vi "Merge Image.vi"(8 "error in (no error)":errorcluster, 10 "Camera Control Cluster":T1={"Core"={"Current VI Reference"=refnum, "Close Panel on Exit?"=FALSE}, "CC ID"=0, "Part name"="", "Number of active cameras"=[], "IA Camera names"=[], "Image count array"=[], "Diagnostics Child ID"=-1, "Number of cameras"=0, "Image array"=[], "LiveMode"=TRUE, "RecieversID"=[], "Active Camera ID"=[], "Enqueuer"={"Caller Enqueuer"=refnum, "Nested Actor's Enqueuer"=[], "Reciever Enqueuer "=[]}, "Image Array Counter"=0, "Images Recieved count"=[], "All Camera Diagnostics"=FALSE, "Output Data"={"Launch Handshake"={"Actor Enqueuer Refnum"=refnum, "Actor core Refnum"=refnum, "Actor Name"=""}, "Launch Clear"=TRUE, "Part Name"="", "Image Trigger Count"=0, "Image Array"=[], "CamOpticsDiagnosticsResult"={"Light Camera  Name"="", "Diagnosed Image"=refnum, "Dust Percentage"=0.0, "Result"=FALSE}, "State Ack"={"State Message"="", "Status"=""}, "Error Handler"="", "Camera Information"=[], "Number of Active Camera"=0}, "Camera Setup"=[], "Setup Response Received Count"=0, "Send Error to Caller"=FALSE, "Camera Info Recieved"=0, "CameraControllerParameters"={"CameraControllerParameters"={"ID"=0, "FrontPanelOpen"=FALSE, "NoOfCameras"=0, "CameraID"=[], "NoOfReceivers"=0, "Diagnostics"={"Path"="", "LightCameraSequence"=[], "Delaytime"=0.0, "DecisitionParameters"={"Range"=[], "AcceptancePercentage"=[], "Comparison"=[], "AcceptableBlackBinValue"=0}, "DiagnosticReceiverSequence"={"ReceiverName"="", "ReceiverID"=0}}, "PartsList"=[]}, "PartName"=[]}, "CurrentPartDetails"={"PartName"="", "CameraIDs"=[], "ReceiverSequence"=[]}, "Run Info"={"State"="", "Image File path"=[]}, "Active Light Camera Name"="", "Captured Image Info"={"Image out"=refnum, "Camera Location"="", "Count"=0, "RecieverSequence"=[{"RecieverID"=0.0, "Index"=1.0}, {"RecieverID"=1.0, "Index"=2.0}]}, "Current Steps"="", "CurrentReceiverSequence"=[], "Status Ack"=[]}, 11 "Camera Controller in":refnum<class "Camera Controller.lvclass">) -> (0 "error out":errorcluster, 2 "Camera Control Cluster Out":T1={"Core"={"Current VI Reference"=refnum, "Close Panel on Exit?"=FALSE}, "CC ID"=0, "Part name"="", "Number of active cameras"=[], "IA Camera names"=[], "Image count array"=[], "Diagnostics Child ID"=-1, "Number of cameras"=0, "Image array"=[], "LiveMode"=TRUE, "RecieversID"=[], "Active Camera ID"=[], "Enqueuer"={"Caller Enqueuer"=refnum, "Nested Actor's Enqueuer"=[], "Reciever Enqueuer "=[]}, "Image Array Counter"=0, "Images Recieved count"=[], "All Camera Diagnostics"=FALSE, "Output Data"={"Launch Handshake"={"Actor Enqueuer Refnum"=refnum, "Actor core Refnum"=refnum, "Actor Name"=""}, "Launch Clear"=TRUE, "Part Name"="", "Image Trigger Count"=0, "Image Array"=[], "CamOpticsDiagnosticsResult"={"Light Camera  Name"="", "Diagnosed Image"=refnum, "Dust Percentage"=0.0, "Result"=FALSE}, "State Ack"={"State Message"="", "Status"=""}, "Error Handler"="", "Camera Information"=[], "Number of Active Camera"=0}, "Camera Setup"=[], "Setup Response Received Count"=0, "Send Error to Caller"=FALSE, "Camera Info Recieved"=0, "CameraControllerParameters"={"CameraControllerParameters"={"ID"=0, "FrontPanelOpen"=FALSE, "NoOfCameras"=0, "CameraID"=[], "NoOfReceivers"=0, "Diagnostics"={"Path"="", "LightCameraSequence"=[], "Delaytime"=0.0, "DecisitionParameters"={"Range"=[], "AcceptancePercentage"=[], "Comparison"=[], "AcceptableBlackBinValue"=0}, "DiagnosticReceiverSequence"={"ReceiverName"="", "ReceiverID"=0}}, "PartsList"=[]}, "PartName"=[]}, "CurrentPartDetails"={"PartName"="", "CameraIDs"=[], "ReceiverSequence"=[]}, "Run Info"={"State"="", "Image File path"=[]}, "Active Light Camera Name"="", "Captured Image Info"={"Image out"=refnum, "Camera Location"="", "Count"=0, "RecieverSequence"=[{"RecieverID"=0.0, "Index"=1.0}, {"RecieverID"=1.0, "Index"=2.0}]}, "Current Steps"="", "CurrentReceiverSequence"=[], "Status Ack"=[]}, 3 "Camera Controller out":refnum<class "Camera Controller.lvclass">)   [LabVIEW 2019, in "Camera Controller.lvlib" / "Camera Controller.lvclass"]
uses:
  Camera Controller.lvclass
  <vilib>/vision/Image Controls.llb/IMAQ Image.ctl
  <vilib>/ActorFramework/Actor/Actor.lvclass
  Image Trigger Global Count.vi
  C:/Program Files/National Instruments/LabVIEW 2019/vi.lib/ActorFramework/Actor/Actor.lvclass
  <vilib>/ActorFramework/Message Enqueuer/Message Enqueuer.lvclass
  TypeDef/Output Data.ctl
  TypeDef/CameraControllerParameters.ctl
  TypeDef/Initialize Data CC.ctl
panel:
  out "min value":i32
  out "output array":T2[][](array[typedef])
  in  "appended array in":T2[][](array[typedef])
  out "appended array out":T2[][](array[typedef])
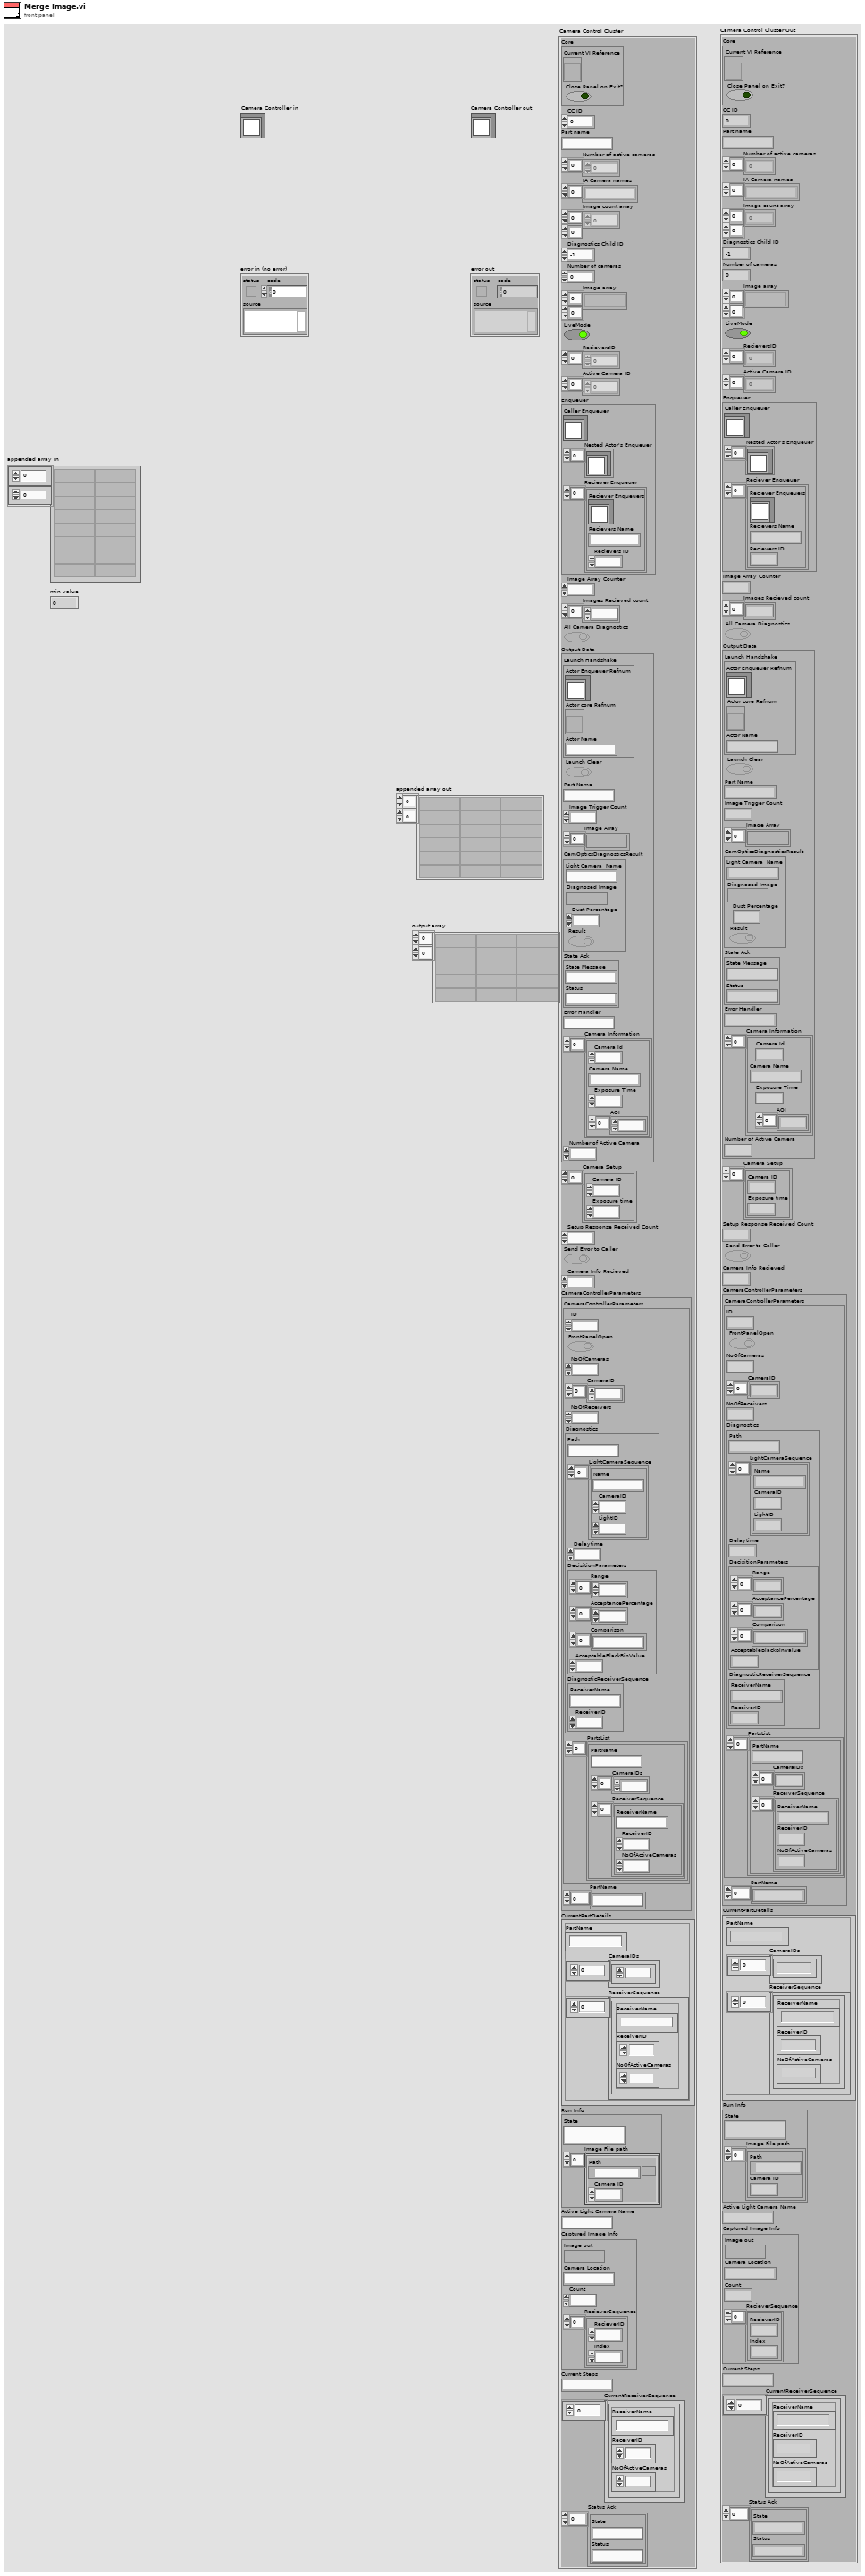
[diagram p1: front panel]
types:
  T1 = typedef "Camera Controller.lvlib/Camera Controller.lvclass/Initialize Data CC.ctl" = cluster{"Core":cluster{"Current VI Reference":refnum<vi>, "Close Panel on Exit?":bool}, "CC ID":i32, "Part name":string, "Number of active cameras":i32[], "IA Camera names":string[], "Image count array":i32[][], "Diagnostics Child ID":i32, "Number of cameras":i32, "Image array":T2[][], "LiveMode":bool, "RecieversID":i32[], "Active Camera ID":i32[], "Enqueuer":cluster{"Caller Enqueuer":refnum<class "Message Enqueuer.lvclass">, "Nested Actor's Enqueuer":refnum<class "Message Enqueuer.lvclass">[], "Reciever Enqueuer ":cluster{"Reciever Enqueuers":refnum<class "Message Enqueuer.lvclass">, "Recievers Name":string, "Recievers ID":i32}[]}, "Image Array Counter":u64, "Images Recieved count":u64[], "All Camera Diagnostics":bool, "Output Data":T3, "Camera Setup":cluster{"Camera ID":i32, "Exposure time":i32}[], "Setup Response Received Count":u64, "Send Error to Caller":bool, "Camera Info Recieved":i32, "CameraControllerParameters":T4, "CurrentPartDetails":cluster{"PartName":string, "CameraIDs":i32[], "ReceiverSequence":cluster{"ReceiverName":string, "ReceiverID":i32, "NoOfActiveCameras":i32}[]}, "Run Info":cluster{"State":string, "Image File path":cluster{"Path":path, "Camera ID":i32}[]}, "Active Light Camera Name":string, "Captured Image Info":cluster{"Image out":T2, "Camera Location":string, "Count":u64, "RecieverSequence":cluster{"RecieverID":dbl, "Index":dbl}[]}, "Current Steps":string, "CurrentReceiverSequence":cluster{"ReceiverName":string, "ReceiverID":i32, "NoOfActiveCameras":i32}[], "Status Ack":cluster{"State":string, "Status":string}[]}
  T2 = typedef "IMAQ Image.ctl" = refnum<image>
  T3 = typedef "Camera Controller.lvlib/Camera Controller.lvclass/Output Data.ctl" = cluster{"Launch Handshake":cluster{"Actor Enqueuer Refnum":refnum<class "Message Enqueuer.lvclass">, "Actor core Refnum":refnum<vi>, "Actor Name":string}, "Launch Clear":bool, "Part Name":string, "Image Trigger Count":u64, "Image Array":T2[], "CamOpticsDiagnosticsResult":cluster{"Light Camera  Name":string, "Diagnosed Image":T2, "Dust Percentage":dbl, "Result":bool}, "State Ack":cluster{"State Message":string, "Status":string}, "Error Handler":string, "Camera Information":cluster{"Camera Id":i32, "Camera Name":string, "Exposure Time":i32, "AOI":i32[]}[], "Number of Active Camera":i32}
  T4 = typedef "Camera Controller.lvlib/Camera Controller.lvclass/CameraControllerParameters.ctl" = cluster{"CameraControllerParameters":cluster{"ID":i32, "FrontPanelOpen":bool, "NoOfCameras":i32, "CameraID":i32[], "NoOfReceivers":i32, "Diagnostics":cluster{"Path":string, "LightCameraSequence":cluster{"Name":string, "CameraID":i32, "LightID":i32}[], "Delaytime":dbl, "DecisitionParameters":cluster{"Range":i32[], "AcceptancePercentage":i32[], "Comparison":string[], "AcceptableBlackBinValue":i32}, "DiagnosticReceiverSequence":cluster{"ReceiverName":string, "ReceiverID":i32}}, "PartsList":cluster{"PartName":string, "CameraIDs":i32[], "ReceiverSequence":cluster{"ReceiverName":string, "ReceiverID":i32, "NoOfActiveCameras":i32}[]}[]}, "PartName":string[]}
  T5 = cluster{"ReceiverName":string, "ReceiverID":i32, "NoOfActiveCameras":i32}[]
  T6 = cluster{"ReceiverName":string, "ReceiverID":i32, "NoOfActiveCameras":i32}
  T7 = cluster{"Reciever Enqueuers":refnum<class "Message Enqueuer.lvclass">, "Recievers Name":string, "Recievers ID":i32}[]
  T8 = cluster{"Reciever Enqueuers":refnum<class "Message Enqueuer.lvclass">, "Recievers Name":string, "Recievers ID":i32}
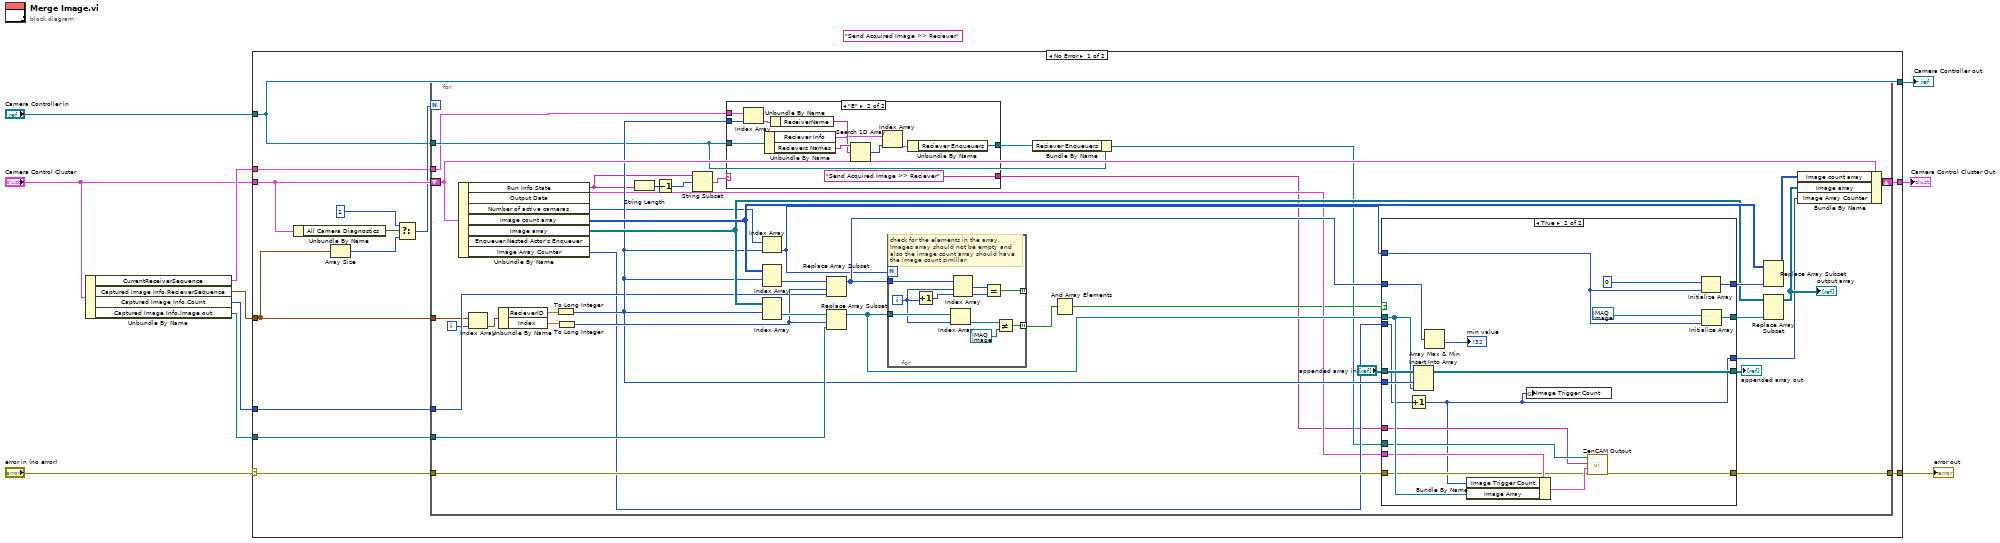
[diagram p0: block diagram]
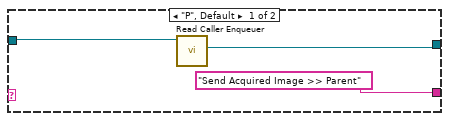
[diagram p2: hidden frame]
diagram:
  (unwired) "Send Acquired Image >> Reciever" ("State")
  n1 = Unbundle By Name("Camera Control Cluster") -> ("CurrentReceiverSequence"=w8:T5, "Captured Image Info.RecieverSequence"=w7:cluster{"RecieverID":dbl, "Index":dbl}[], "Captured Image Info.Count"=w6:u64, "Captured Image Info.Image out"=w5:T2)
  n2 = case shown="No Error" "error in (no error)" {
    selector: "error in (no error)" -> [w21 w114]
    tunnel: w7 -> [w17 _]
    tunnel: w6 -> [w23 _]
    tunnel: w5 -> [w15 _]
    tunnel: "Camera Control Cluster" -> [w19 w115]
    tunnel: [w22 w115] -> w2
    tunnel: [w20 w114] -> w3
    tunnel: w8 -> [w12 _]
    tunnel: "Camera Controller in" -> [w11 w113]
    tunnel: [w11 w113] -> w1
    frame No Error {
      n3 = Unbundle By Name(w19) -> ("All Camera Diagnostics"=w16:bool)
      n4 = Array Size(array=w17) -> (size(s)=w13:i32)
      n5 = Select(t=1 ("f"), s=w16, f=w13) -> (s? t:f=w18:i32)
      n6 = for {
        N: w18 -> [_]
        tunnel: w23 -> [w44]
        tunnel: w15 -> [w59]
        shift-right: [w50] -> w22
        shift-left: w19 -> [w57]
        tunnel: w21 -> [w45]
        tunnel: [w46] -> w20
        tunnel: w17 -> [w36]
        tunnel: w12 -> [w25]
        tunnel: w11 -> [w33]
        i -> [w37]
        n7 = Unbundle By Name(w57) -> ("Run Info.State"=w27:string, "Output Data"=w34:T3, "Number of active cameras"=w43:i32[], "Image count array"=w54:i32[][], "Image array"=w53:T2[][], "Image Array Counter"=w39:u64)  [unwired: 1 out]
        n8 = Index Array(array=w36, index=w37) -> (element=w35:cluster{"RecieverID":dbl, "Index":dbl})
        n9 = Unbundle By Name(w35) -> ("RecieverID"=w64:dbl, "Index"=w63:dbl)
        n10 = To Long Integer(number=w64) -> (32bit integer=w48:i32)
        n11 = To Long Integer(number=w63) -> (32bit integer=w60:i32)
        n12 = String Length(string=w27) -> (length=w29:i32)
        n13 = Decrement(x=w29) -> (x-1=w28:i32)
        n14 = String Subset(string=w27, offset (0)=w28) -> (substring=w26:string)  [unwired: 1 in]
        n15 = case shown="\"E\"" w26 {
          tunnel: w48 -> [_ w78]
          tunnel: w25 -> [_ w77]
          tunnel: w33 -> [w67 w71]
          tunnel: [w66 w69] -> w32
          tunnel: ["Send Acquired Image >> Parent" ("State") "Send Acquired Image >> Reciever" ("State")] -> w24
          frame "P", Default {
            n16 = call <vilib>:"Read Caller Enqueuer.vi"("Actor"=w67) -> ("Caller Enqueuer"=w66:refnum<class "Message Enqueuer.lvclass">)  [unwired: 10 in]
          }
          frame "E" {
            n17 = Index Array(array=w77, index=w78) -> (element=w76:T6)
            n18 = Unbundle By Name(w71) -> ("Reciever Info"=w73:T7, "Recievers Names"=w75:string[])
            n19 = Unbundle By Name(w76) -> ("ReceiverName"=w74:string)
            n20 = Search 1D Array(1D array=w75, element=w74) -> (index of element=w72:i32)  [unwired: 1 in]
            n21 = Index Array(array=w73, index=w72) -> (element=w70:T8)
            n22 = Unbundle By Name(w70) -> ("Reciever Enqueuers"=w69:refnum<class "Message Enqueuer.lvclass">)
          }
        }
        n23 = Index Array(array=w43, index=w48) -> (element=w41:i32)
        n24 = Index Array(array=w54, index (row)=w48) -> (element=w62:i32[])  [unwired: 1 in]
        n25 = Index Array(array=w53, index (row)=w48) -> (element=w61:T2[])  [unwired: 1 in]
        n26 = Replace Array Subset(array=w62, new element=w44, index=w60) -> (w42:i32[])
        n27 = Replace Array Subset(array=w61, new element=w59, index=w60) -> (w40:T2[])
        n28 = for {
          N: w41 -> [_]
          tunnel: w40 -> [w112]
          tunnel: [w109] -> w58 mode=indexing
          tunnel: w42 -> [w108]
          tunnel: [w104] -> _ mode=indexing
          i -> [w103]
          # "check for the elements in the array, Images array should not be empty and also the image count array should have the image count simillar"
          n29 = Increment(x=w103) -> (x+1=w107:i32)
          n30 = Index Array(array=w112, index=w103) -> (element=w111:T2)
          n31 = Index Array(array=w108, index #1=w103, index #2=w107) -> (element #1=w106:i32, element #2=w105:i32)
          n32 = Equal?(x=w106, y=w105) -> (x = y?=w104:bool)
          n33 = Not Equal?(x=w111, y=T2 refnum) -> (x != y?=w109:bool)
        }
        n34 = Bundle By Name(cluster=w33, "Reciever Enqueuers"=w32) -> (w31:refnum<class "Camera Controller.lvclass">)
        n35 = And Array Elements(Boolean array=w58) -> (logical AND=w30:bool)
        n36 = case shown="True" w30 {
          tunnel: w40 -> [w82 w92]
          tunnel: w42 -> [w83 w93]
          tunnel: w41 -> [_ w98]
          tunnel: [w83 w100] -> w56
          tunnel: [w82 w99] -> w55
          tunnel: "appended array in" -> [w81 w97]
          tunnel: w48 -> [_ w95]
          tunnel: [w81 w96] -> w47
          tunnel: w45 -> [w80 w85]
          tunnel: [w80 w94] -> w46
          tunnel: w39 -> [w79 w90]
          tunnel: [w79 w84] -> w38
          tunnel: w34 -> [_ w89]
          tunnel: w31 -> [_ w88]
          tunnel: w24 -> [_ w86]
          frame False {
          }
          frame True {
            n37 = Increment(x=w90) -> (x+1=w84:u64)
            n38 = Insert Into Array(array=w97, index (col)=w95, new element=w92) -> (w96:T2[][])  [unwired: 1 in]
            n39 = Array Max & Min(array=w93) -> (min value=→"min value":i32)  [unwired: 3 out]
            n40 = Bundle By Name(cluster=w89, "Image Trigger Count"=w84, "Image Array"=w92) -> (w87:T3)
            n41 = global write "Image Trigger Global Count.vi" "Image Trigger Count"(w84) -> ()
            n42 = call "ZenCAM Output.vi"("error in (no error)"=w85, "Output Data"=w87, "State"=w86, "Camera Controller in"=w88) -> ("error out"=w94:errorcluster)  [unwired: 6 in, 1 out]
            n43 = Initialize Array(0, w98) -> (w100:i32[])
            n44 = Initialize Array(T2 refnum ("y"), w98) -> (w99:T2[])
          }
        }
        "appended array out" <- w47
        n45 = Replace Array Subset(array=w54, new element=w56) -> (w52:i32[][])  [unwired: 2 in]
        n46 = Replace Array Subset(array=w53, new element=w55) -> (w51:T2[][])  [unwired: 2 in]
        "output array" <- w51
        n47 = Bundle By Name(cluster=w57, "Image count array"=w52, "Image array"=w51, "Image Array Counter"=w38) -> (w50:T1)
      }
    }
    frame Error {
    }
  }
  "error out" <- w3
  "Camera Controller out" <- w1
  "Camera Control Cluster Out" <- w2
